vi "serial_p_p (SubVI).vi"(9 "Command":string, 10 "delay before read (ms)":u32=500, 11 "VISA Refnum in":refnum<visa-resource-name>) -> (0 "error out":errorcluster, 2 "read buffer":string, 3 "VISA Refnum out":refnum<visa-resource-name>)   [LabVIEW 2013]
uses:
  <vilib>/Instr/_visa.llb/VISA Configure Serial Port (Instr).vi
panel:
  out "length":i32
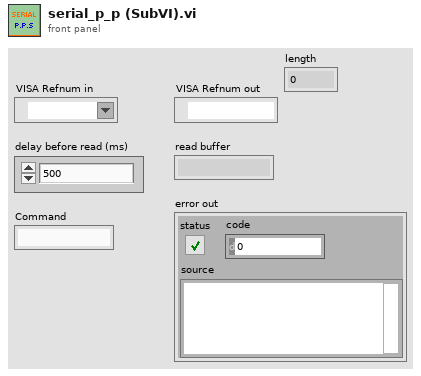
[diagram p1: front panel]
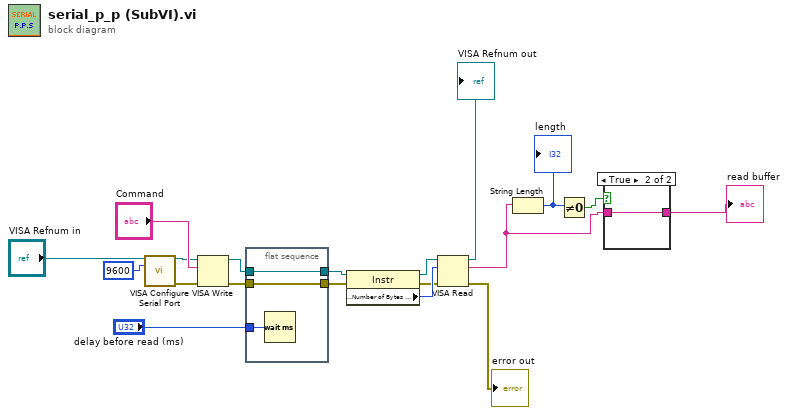
[diagram p0: block diagram]
diagram:
  n1 = call-poly "VISA Configure Serial Port"("VISA resource name"="VISA Refnum in", "baud rate (9600)"=u32 9600) -> ("VISA resource name out"=w8:refnum<visa-resource-name>, "error out"=w7:errorcluster)  [unwired: 7 in, 5 out]
  n2 = VISA Write(VISA resource name=w8, write buffer="Command", error in (no error)=w7) -> (VISA resource name out=w13:refnum<visa-resource-name>, error out=w11:errorcluster)  [unwired: 1 out]
  n3 = flat-sequence {
    tunnel: w11 -> [w21]
    tunnel: [w21] -> w12
    tunnel: w13 -> [w20]
    tunnel: [w20] -> w14
    tunnel: "delay before read (ms)" -> [w22]
    frame #0 {
      n4 = Wait (ms)(milliseconds to wait=w22) -> ()  [unwired: 1 out]
    }
  }
  n5 = property class="Instr"(reference=w14, error in=w12) -> (reference out=w17:refnum<visa-resource-name>, error out=w18:errorcluster, "Serial Settings:Number of Bytes at Serial Port"=w19:u32)
  n6 = VISA Read(VISA resource name=w17, byte count=w19, error in (no error)=w18) -> (VISA resource name out=→"VISA Refnum out":refnum<visa-resource-name>, read buffer=w1:string, error out=→"error out":errorcluster)  [unwired: 1 out]
  n7 = String Length(string=w1) -> (length=w3:i32)
  "length" <- w3
  n8 = Not Equal To 0?(x=w3) -> (x != 0?=w2:bool)
  n9 = case shown="True" w2 {
    tunnel: [_ w23] -> w4
    tunnel: w1 -> [_ w23]
    frame False {
    }
    frame True {
    }
  }
  "read buffer" <- w4
